vi "SetInitialControlValues.vi"(8 "error in (no error)":errorcluster, 10 "ControlValueUpdates[] in":T1[](array[typedef]), 11 "UI_Interaction_Manager in":refnum<class "UI_Interaction_Manager.lvclass">) -> (0 "error out":errorcluster, 2 "ControlValueUpdates[] out":T1[](array[typedef]), 3 "UI_Interaction_Manager out":refnum<class "UI_Interaction_Manager.lvclass">)   [LabVIEW 2011, in "UI_Interaction_Manager.lvclass"]
uses:
  UI_Interaction_Manager.lvclass
  TypeDefs/ControlValueUpdate.ctl
  UI_Interaction_Manager.lvclass/UI_Interaction_Manager.ctl
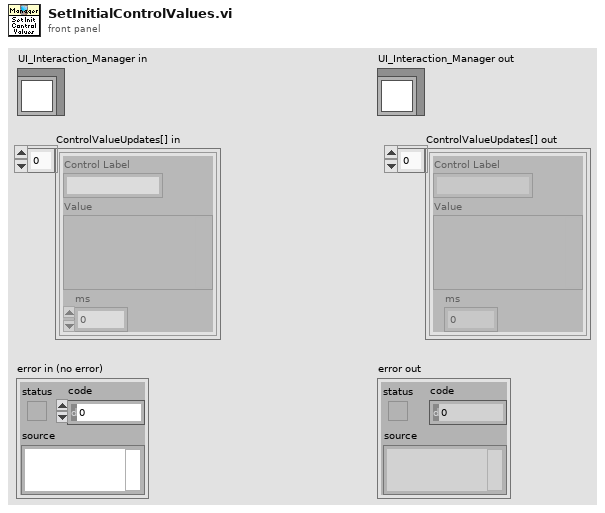
[diagram p1: front panel]
types:
  T1 = typedef "UI_Interaction_Manager.lvclass/ControlValueUpdate.ctl" = cluster{"Control Label":string, "Value":variant, "ms":u32}
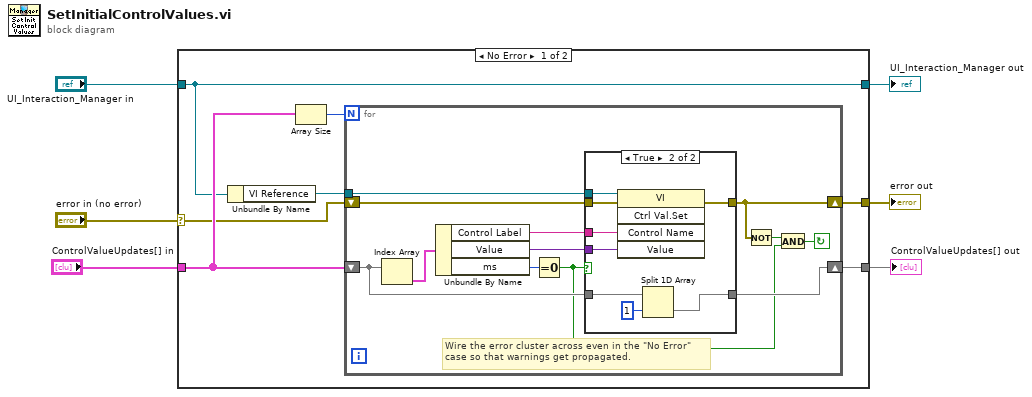
[diagram p0: block diagram]
diagram:
  n1 = case shown="No Error" "error in (no error)" {
    selector: "error in (no error)" -> [w10 w37]
    tunnel: [w9 w37] -> w5
    tunnel: [w11 w36] -> w3
    tunnel: "UI_Interaction_Manager in" -> [w11 w36]
    tunnel: "ControlValueUpdates[] in" -> [w12 _]
    tunnel: [w7 _] -> w1
    frame No Error {
      # "Wire the error cluster across even in the \"No Error\"\ncase so that warnings get propagated."
      n2 = Unbundle By Name(w11) -> ("VI Reference"=w8:refnum<vi>)
      n3 = Array Size(array=w12) -> (size(s)=w13:i32)
      n4 = for {
        N: w13 -> [_]
        shift-right: [w20] -> w7
        shift-left: w12 -> [w21]
        shift-right: [w18] -> w9
        shift-left: w10 -> [w19]
        tunnel: w8 -> [w14]
        stop <- w15 continue-if-true
        n5 = Index Array(array=w21) -> (element=w22:T1)  [unwired: 1 in]
        n6 = Unbundle By Name(w22) -> ("Control Label"=w25:string, "Value"=w24:variant, "ms"=w23:u32)
        n7 = Equal To 0?(x=w23) -> (x = 0?=w16:bool)
        n8 = case shown="True" w16 {
          tunnel: w14 -> [_ w35]
          tunnel: w25 -> [_ w34]
          tunnel: w24 -> [_ w33]
          tunnel: w21 -> [w27 w32]
          tunnel: [w27 w30] -> w20
          tunnel: w19 -> [w26 w29]
          tunnel: [w26 w28] -> w18
          frame False {
          }
          frame True {
            n9 = invoke class="VI" method="Ctrl Val.Set"(reference=w35, error in=w29, "Control Name"=w34, "Value"=w33) -> (error out=w28:errorcluster)  [unwired: 1 in, 4 out]
            n10 = Split 1D Array(array=w32, index=1) -> (second subarray=w30:T1[])  [unwired: 1 out]
          }
        }
        n11 = Not(x=w18) -> (.not. x?=w17:bool)
        n12 = And(x=w17, y=w16) -> (x .and. y?=w15:bool)
      }
    }
    frame Error {
    }
  }
  "error out" <- w5
  "UI_Interaction_Manager out" <- w3
  "ControlValueUpdates[] out" <- w1
